vi "Is Variable Name Part of Struct.vi"(11 "variable name":string) -> (3 "Is part of struct?":bool)   [LabVIEW 2013, in "GOLPI library.lvlib"]
doc: "Checks if variable name is part of structure. Tests for dots in the variable name. 'A.B' results in True, 'AB' results in False. This is because some functions can have problems operating with variable names composed of Structure.Something."
uses:
  GOLPI library.lvlib
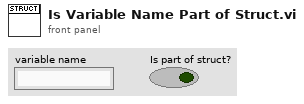
[diagram p1: front panel]
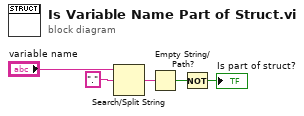
[diagram p0: block diagram]
diagram:
  n1 = Search/Split String(string="variable name", search string/char (-)=".") -> (match + rest of string=w4:string)  [unwired: 1 in, 2 out]
  n2 = Empty String/Path?(string/path=w4) -> (empty?=w2:bool)
  n3 = Not(x=w2) -> (.not. x?=→"Is part of struct?":bool)
